vi "Panel Resized.vi"(6 "Sizing Refnums":T2, 8 "error in (no error)":errorcluster, 9 "Origin":cluster{"H":i16, "V":i16}, 10 "NewBnds":T1, 11 "Size Constraints":cluster{"min tab width":i32, "w/h":dbl}) -> (0 "error out":errorcluster)   [LabVIEW 2014]
uses:
  <vilib>/Utility/miscctls.llb/LVRectTypeDef.ctl
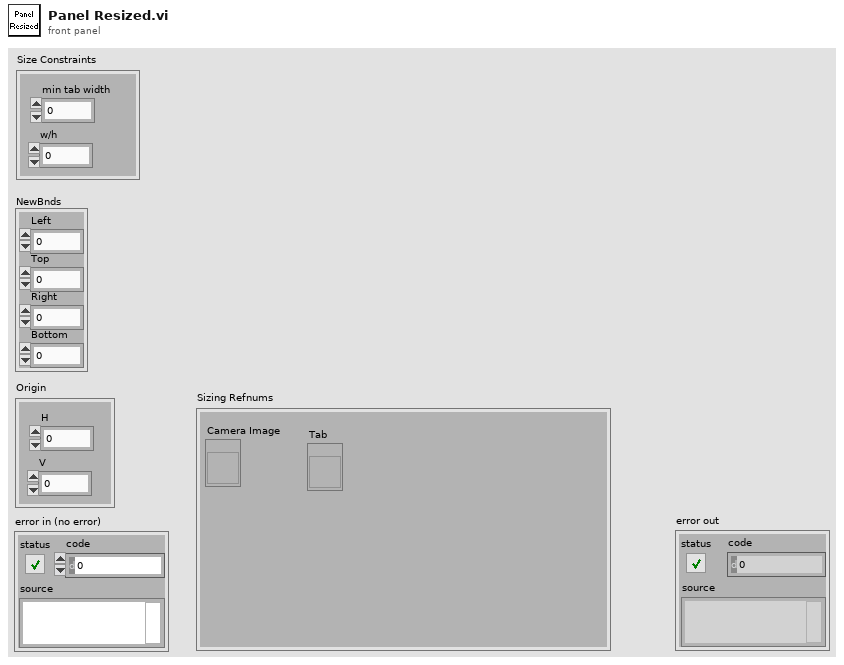
[diagram p1: front panel]
types:
  T1 = typedef "LVRectTypeDef.ctl" = cluster{"Left":i16, "Top":i16, "Right":i16, "Bottom":i16}
  T2 = cluster{"Camera Image":refnum<vi>, "Tab":refnum<vi>}
  T3 = typedef "LVPositionTypeDef.ctl" = cluster{"Left":i32, "Top":i32}
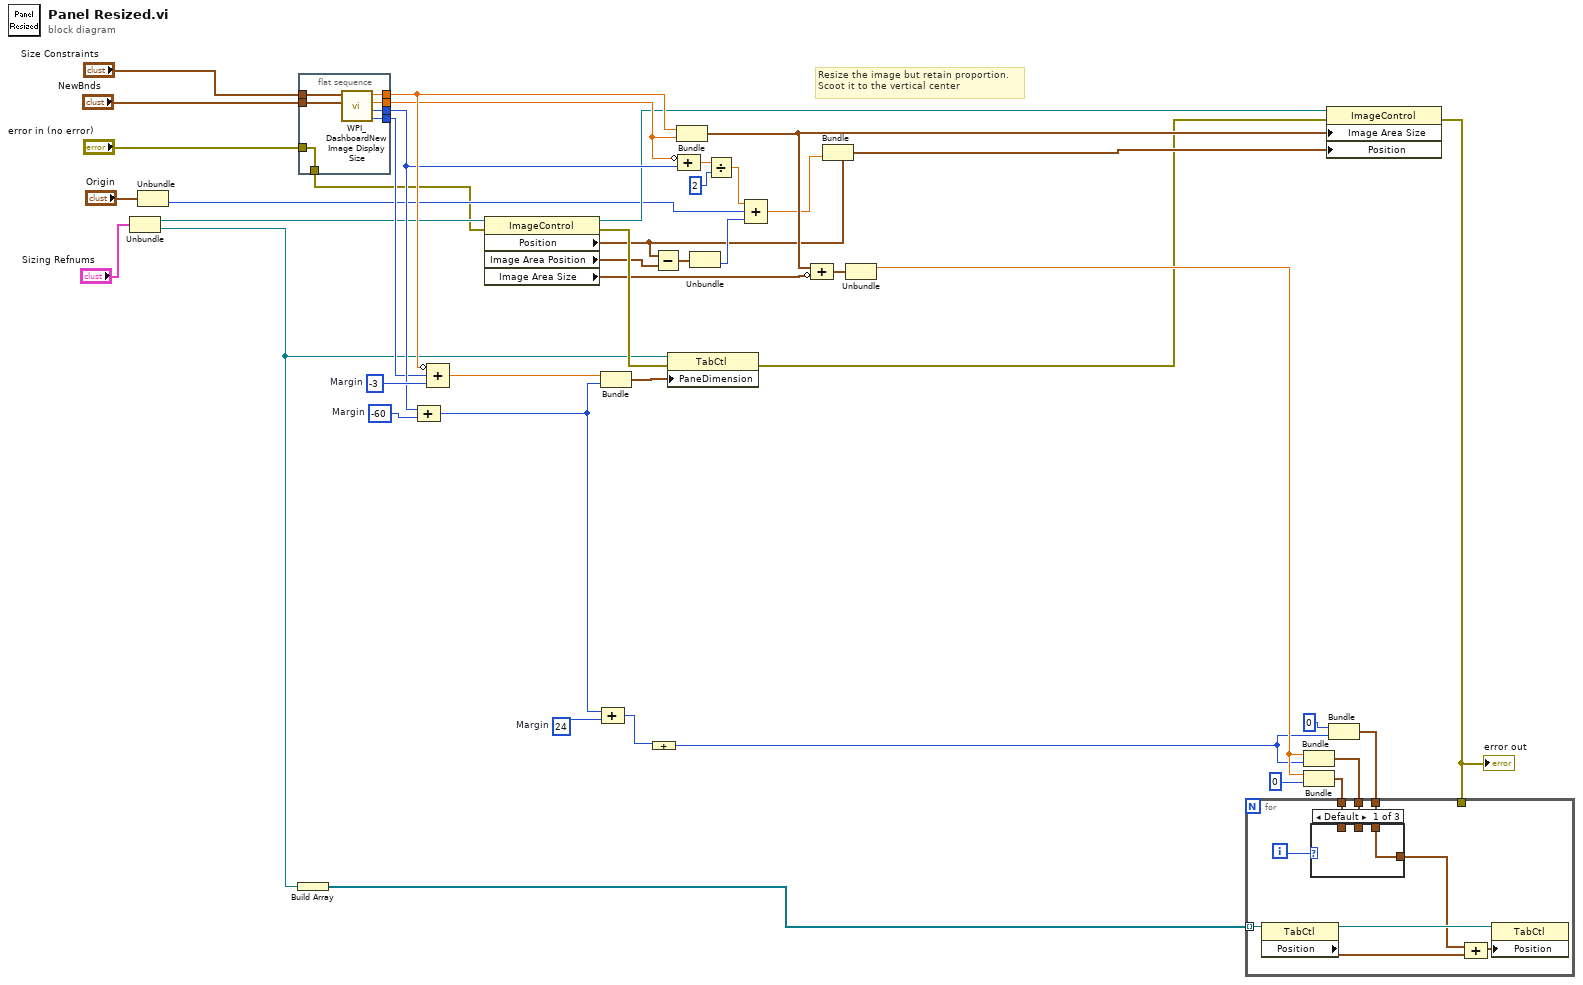
[diagram p0: block diagram]
diagram:
  w35 = 24  # Margin
  w32 = -60  # Margin
  w39 = -3  # Margin
  # "Resize the image but retain proportion.\nScoot it to the vertical center"
  n1 = Unbundle("Sizing Refnums") -> ("Camera Image"=w7:refnum<vi>, "Tab"=w8:refnum<vi>)
  n2 = Unbundle("Origin") -> ("V"=w13:i16)  [unwired: 1 out]
  n3 = Build Array(w8) -> (w44:refnum<vi>[])
  n4 = flat-sequence {
    tunnel: "NewBnds" -> [w51]
    tunnel: "Size Constraints" -> [w50]
    tunnel: [w49] -> w31
    tunnel: [w48] -> w36
    tunnel: [w47] -> w37
    tunnel: [w46] -> w38
    tunnel: [w45] -> w2
    tunnel: "error in (no error)" -> [w45]
    frame #0 {
      n5 = call <vilib>:"WPI_DashboardNew Image Display Size.vi"("NewBnds"=w51, "Size Constraints"=w50) -> ("Window Width"=w49:i16, "Window Height"=w47:i16, "Height"=w48:dbl, "Width"=w46:dbl)  [unwired: 6 in]
    }
  }
  n6 = Compound Arithmetic op=unknown(w37, w32) -> (w34:i32)
  n7 = Compound Arithmetic op=ADD(invert w38, w31, w39) -> (w33:dbl)
  n8 = property class="ImageControl"(reference=w7, error in=w2) -> (reference out=w24:refnum<vi>, error out=w43:errorcluster, "Position"=w23:T3, "Image Area Position"=w18:cluster{"Left":i32, "Top":i32}, "Image Area Size"=w29:cluster{"Width":u32, "Height":u32})
  n9 = Bundle(w33, w34) -> (w6:cluster{dbl, i32})  [unwired: 1 in]
  n10 = Compound Arithmetic op=ADD(w34, w35) -> (w40:i32)
  n11 = Subtract(x=w23, y=w18) -> (x-y=w25:T3)
  n12 = Compound Arithmetic op=ADD(w40) -> (w5:i32)
  n13 = property class="TabCtl"(reference=w8, error in=w43, "PaneDimension"=w6) -> (error out=w1:errorcluster)  [unwired: 1 out]
  n14 = Bundle("Width"=w38, "Height"=w36) -> (w27:cluster{"Width":dbl, "Height":dbl})  [unwired: 1 in]
  n15 = Compound Arithmetic op=ADD(invert w36, w37) -> (w19:dbl)
  n16 = Unbundle(w25) -> ("Top"=w26:i32)  [unwired: 1 out]
  n17 = Divide(x=w19, y=2) -> (x/y=w21:dbl)
  n18 = Compound Arithmetic op=ADD(w21, w13, w26) -> (w22:dbl)
  n19 = Compound Arithmetic op=ADD(w27, invert w29) -> (w30:cluster{"Width":dbl, "Height":dbl})
  n20 = Bundle(cluster=w23, "Top"=w22) -> (w28:T3)  [unwired: 1 in]
  n21 = Unbundle(w30) -> ("Width"=w41:dbl)  [unwired: 1 out]
  n22 = Bundle("Width"=w41, w5) -> (w17:cluster{"Width":dbl, i32})  [unwired: 1 in]
  n23 = Bundle("Width"=w41, 0) -> (w16:cluster{"Width":dbl, i32})  [unwired: 1 in]
  n24 = property class="ImageControl"(reference=w24, error in=w1, "Image Area Size"=w27, "Position"=w28) -> (error out=w12:errorcluster)  [unwired: 1 out]
  "error out" <- w12
  n25 = Bundle(0, w5) -> (w3:cluster{i32, i32})  [unwired: 1 in]
  n26 = for {
    tunnel: w44 -> [w60] mode=indexing
    tunnel: w17 -> [w54]
    tunnel: w16 -> [w55]
    tunnel: w12 -> [_]
    tunnel: w3 -> [w53]
    i -> [w56]
    n27 = property class="TabCtl"(reference=w60) -> (reference out=w59:refnum<vi>, "Position"=w58:T3)  [unwired: 1 in, 1 out]
    n28 = case shown="Default" w56 {
      tunnel: w55 -> [_ w62 _]
      tunnel: w54 -> [_ _ w63]
      tunnel: w53 -> [w61 _ _]
      tunnel: [w61 w62 w63] -> w52
      frame Default {
      }
      frame 0, 1 {
      }
      frame 2, 3 {
      }
    }
    n29 = Compound Arithmetic op=ADD(w52, w58) -> (w57:cluster{dbl, i32})
    n30 = property class="TabCtl"(reference=w59, "Position"=w57) -> ()  [unwired: 1 in, 2 out]
  }
